vi "K2000_get_array.vi"(2 "samples":u16=4096, 3 "address string":string) -> (0 "error out":errorcluster, 1 "Array":sgl[](array[numeric]))   [LabVIEW 2013]
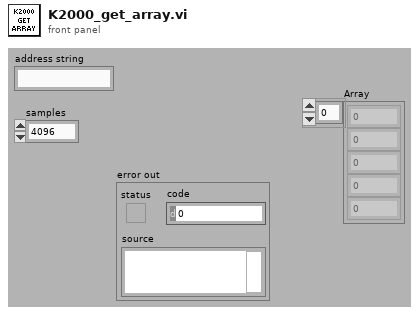
[diagram p1: front panel]
types:
  T1 = enum16{"big-endian, network order", "native, host order", "little-endian"}
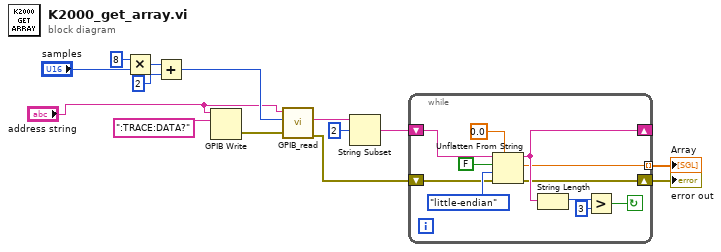
[diagram p0: block diagram]
diagram:
  n1 = Multiply(x=u16 8, y="samples") -> (x*y=w14:u16)
  n2 = Add(x=w14, y=u16 2) -> (x+y=w12:u16)
  n3 = GPIB Write(0:"address string", 1:":TRACE:DATA?" ("data")) -> (6:w8:errorcluster)  [unwired: 1 in, 3 out]
  n4 = call "GPIB_read.vi"("error out 2"=w8, "bytes"=w12, "GPIB Address"="address string") -> ("error out"=w3:errorcluster, "data"=w7:string)  [unwired: 7 out]
  n5 = String Subset(string=w7, offset (0)=2) -> (substring=w5:string)  [unwired: 1 out]
  n6 = while {
    shift-right: [w22] -> _
    shift-left: w5 -> [w25]
    tunnel: [w18] -> w2 mode=indexing
    shift-right: [w16] -> w4
    shift-left: w3 -> [w15]
    stop <- w19 continue-if-true
    n7 = Unflatten From String(type=sgl 0.0, binary string=w25, data includes array or string size? (T)=FALSE, byte order (0:big-endian, network order)=T1."little-endian", error in (no error)=w15) -> (rest of the binary string=w22:string, value=w18:sgl, error out=w16:errorcluster)
    n8 = String Length(string=w22) -> (length=w21:i32)
    n9 = Greater?(x=w21, y=3) -> (0:w19:bool)
  }
  "Array" <- w2
  "error out" <- w4
